vi "Real Uncertain Zero Finder for Imaginary part equals Zero.vi"(4 "data":variant, 5 "x":dbl) -> (2 "f(x)":dbl)   [LabVIEW 2013]
uses:
  BaesDataTypeDefinition.ctl
panel:
  in  "cluster":T2={"Imaginary or Real Part"=0.0, "Chi Square at Minimum"=0.0, "Extinction ExtinctionUncertainity Size parameter and Number ofS sizes"={"Extinction"=[], "Extinction Uncertainty"=[], "Size parameters"=[], "Number ofSizes"=0.0, "GeometricCrossSection"=[], "Wave Length"=0.0, "SMPS Sizes"=[], "Concentration"=[], "Double Charge Correction"=FALSE, "Extincation Factor"=1.0, "Diameter Factor"=1.0, "Diameter Offset"=0.0, "Extinction Factor Flag"=FALSE, "Diameter Factor Flag"=FALSE, "Diameter Offset Flag"=FALSE, "Sizes"=[], "ExtinctionOrAbsorptionOrScattering"=0}} {"Extinction ExtinctionUncertainity Size parameter and Number ofS sizes"."ExtinctionOrAbsorptionOrScattering" scale=0.0..2.0}
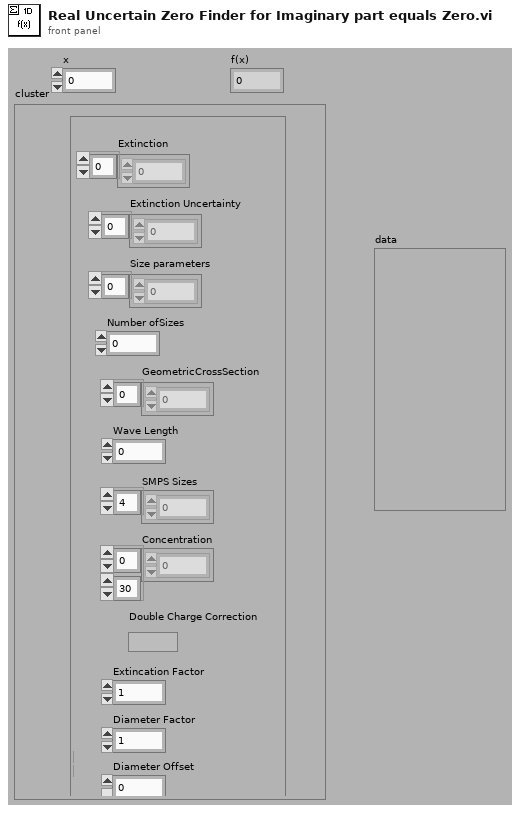
[diagram p1: front panel]
types:
  T1 = typedef "BaesDataTypeDefinition.ctl" = cluster{"Extinction":dbl[], "Extinction Uncertainty":dbl[], "Size parameters":dbl[], "Number ofSizes":dbl, "GeometricCrossSection":dbl[], "Wave Length":dbl, "SMPS Sizes":dbl[], "Concentration":dbl[][], "Double Charge Correction":bool, "Extincation Factor":dbl, "Diameter Factor":dbl, "Diameter Offset":dbl, "Extinction Factor Flag":bool, "Diameter Factor Flag":bool, "Diameter Offset Flag":bool, "Sizes":dbl[], "ExtinctionOrAbsorptionOrScattering":i8}
  T2 = cluster{"Imaginary or Real Part":dbl, "Chi Square at Minimum":dbl, "Extinction ExtinctionUncertainity Size parameter and Number ofS sizes":T1}
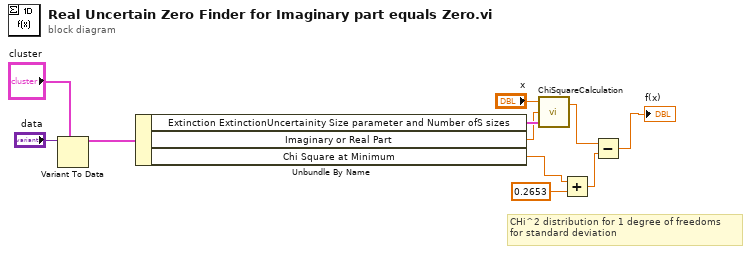
[diagram p0: block diagram]
diagram:
  # "CHi^2 distribution for 1 degree of freedoms\nfor standard deviation"
  n1 = Variant To Data(type="cluster", Variant="data") -> (data=w5:T2)  [unwired: 1 in, 1 out]
  n2 = Unbundle By Name(w5) -> ("Extinction ExtinctionUncertainity Size parameter and Number ofS sizes"=w10:T1, "Imaginary or Real Part"=w9:dbl, "Chi Square at Minimum"=w2:dbl)
  n3 = call "ChiSquareCalculation.vi"("Extinction ExtinctionUncertainity Size parameter and Number ofS sizes 2"=w10, "refractive index, imaginary"=w9, "refractive index, real"="x") -> ("Chi Squared"=w8:dbl)  [unwired: 1 out]
  n4 = Add(x=w2, y=0.2653) -> (x+y=w3:dbl)
  n5 = Subtract(x=w8, y=w3) -> (x-y=→"f(x)":dbl)
